vi "Digital Color Logic.vi"(0 "Sensor Value":dbl=100.0 format="%#_13g", 5 "Thresold Array":dbl[](array[numeric])) -> (4 "Color Out":u32, 6 "Range Max":dbl, 8 "Range Min":dbl, 10 "Span Max":dbl, 15 "Span Min":dbl)   [LabVIEW 2018]
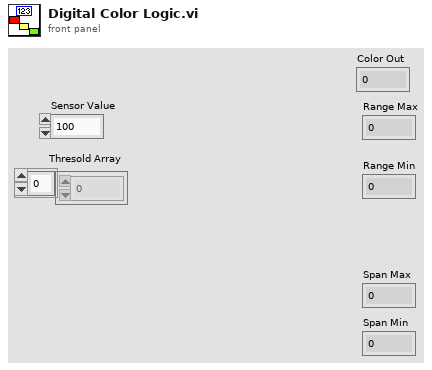
[diagram p1: front panel]
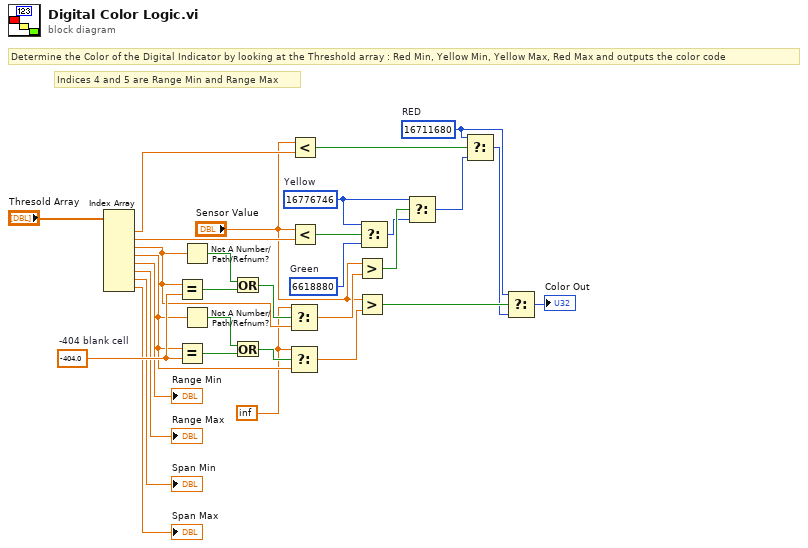
[diagram p0: block diagram]
diagram:
  w1 = inf
  w16 = u32 6618880  # Green
  w14 = u32 16776746  # Yellow
  w23 = u32 16711680  # RED
  w28 = -404.0  # -404 blank cell
  # "Indices 4 and 5 are Range Min and Range Max"
  # "Determine the Color of the Digital Indicator by looking at the Threshold array : Red Min, Yellow Min, Yellow Max, Red Max and outputs the color code"
  n1 = Index Array(array="Thresold Array") -> (element #1=w25:dbl, element #2=w15:dbl, element #3=w7:dbl, element #4=w9:dbl, element #5=→"Range Min":dbl, element #6=→"Range Max":dbl, element #7=→"Span Min":dbl, element #8=→"Span Max":dbl)  [unwired: 8 in]
  n2 = Equal?(x=w7, y=w28) -> (x = y?=w29:bool)
  n3 = Equal?(x=w9, y=w28) -> (x = y?=w30:bool)
  n4 = Not A Number/Path/Refnum?(number/path/refnum=w7) -> (NaN/Path/Refnum?=w6:bool)
  n5 = Not A Number/Path/Refnum?(number/path/refnum=w9) -> (NaN/Path/Refnum?=w10:bool)
  n6 = Or(x=w6, y=w29) -> (x .or. y?=w8:bool)
  n7 = Or(x=w10, y=w30) -> (x .or. y?=w11:bool)
  n8 = Select(t=w1, s=w8, f=w7) -> (s? t:f=w21:dbl)
  n9 = Select(t=w1, s=w11, f=w9) -> (s? t:f=w27:dbl)
  n10 = Less?(x="Sensor Value", y=w25) -> (x < y?=w24:bool)
  n11 = Less?(x="Sensor Value", y=w15) -> (x < y?=w18:bool)
  n12 = Greater?(x="Sensor Value", y=w21) -> (0:w20:bool)
  n13 = Greater?(x="Sensor Value", y=w27) -> (0:w26:bool)
  n14 = Select(t=w14, s=w18, f=w16) -> (s? t:f=w17:u32)
  n15 = Select(t=w14, s=w20, f=w17) -> (s? t:f=w19:u32)
  n16 = Select(t=w23, s=w24, f=w19) -> (s? t:f=w22:u32)
  n17 = Select(t=w23, s=w26, f=w22) -> (s? t:f=→"Color Out":u32)
